vi "Read Fluence Parameter.vi"(11 "Analyze Parameter Fluence in":refnum<class "Analyze Parameter Fluence.lvclass">) -> (0 "#of Areas":i32, 1 "#Overlays":i32, 2 "Size of region (px)":i32, 3 "Analyze Parameter Fluence out":refnum<class "Analyze Parameter Fluence.lvclass">)   [LabVIEW 2020, in "Analyze Parameter Fluence.lvclass"]
uses:
  Analyze Parameter Fluence.lvclass
  Analyze Parameter Fluence.lvclass/Analyze Parameter Fluence.ctl
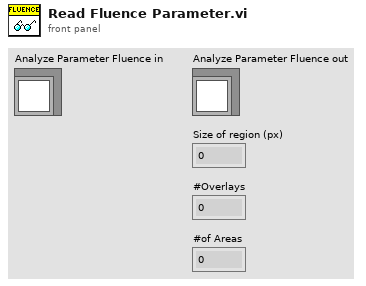
[diagram p1: front panel]
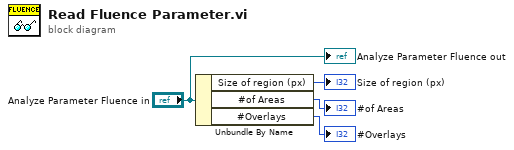
[diagram p0: block diagram]
diagram:
  n1 = Unbundle By Name("Analyze Parameter Fluence in") -> ("Size of region (px)"=→"Size of region (px)":i32, "#of Areas"=→"#of Areas":i32, "#Overlays"=→"#Overlays":i32)
  "Analyze Parameter Fluence out" <- "Analyze Parameter Fluence in"
